vi "util_sort_build_specs.vi"(8 "error in (no error)":errorcluster, 11 "build_specifications in":T1[](array[typedef])) -> (0 "error out":errorcluster, 3 "build_specifications out":T1[](array[typedef]))   [LabVIEW 2015, in "lv-build.lvlib"]
uses:
  lv-build.lvlib
  public/_controls/build_specification.ctl
  public/_controls/build_type.ctl
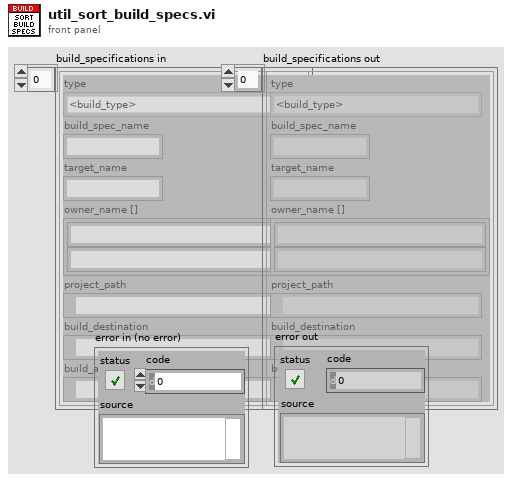
[diagram p1: front panel]
types:
  T1 = typedef "lv-build.lvlib/build_specification.ctl" = cluster{"type":T2, "build_spec_name":string, "target_name":string, "owner_name []":string[], "project_path":path, "build_destination":path, "build_artifact":path}
  T2 = typedef "lv-build.lvlib/build_type.ctl" = enum16{"<build_type>", "application_pc", "application_rt", "installer", "llb", "lvlibp", "zip", "fpga", "<null>"}
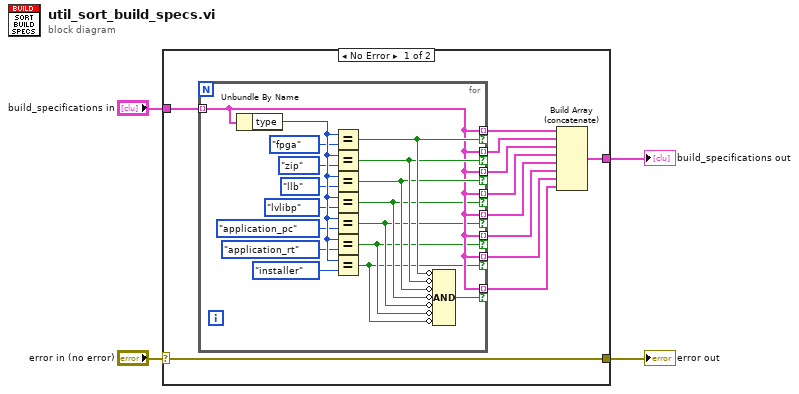
[diagram p0: block diagram]
diagram:
  n1 = case shown="No Error" "error in (no error)" {
    selector: "error in (no error)" -> [w11 w34]
    tunnel: "build_specifications in" -> [w15 w33]
    tunnel: [w12 w33] -> w3
    tunnel: [w11 w34] -> w1
    frame No Error {
      n2 = for {
        tunnel: w15 -> [w28] mode=indexing
        tunnel: [w28] -> w14 mode=indexing if=w31
        tunnel: [w28] -> w5 mode=indexing if=w32
        tunnel: [w28] -> w13 mode=indexing if=w30
        tunnel: [w28] -> w10 mode=indexing if=w29
        tunnel: [w28] -> w9 mode=indexing if=w26
        tunnel: [w28] -> w8 mode=indexing if=w25
        tunnel: [w28] -> w7 mode=indexing if=w24
        tunnel: [w28] -> w6 mode=indexing if=w23
        n3 = Unbundle By Name(w28) -> ("type"=w27:T2)
        n4 = Equal?(x=w27, y=build_type."fpga" ("Type")) -> (x = y?=w31:bool)
        n5 = Equal?(x=w27, y=build_type."zip" ("Type")) -> (x = y?=w30:bool)
        n6 = Equal?(x=w27, y=build_type."llb" ("Type")) -> (x = y?=w29:bool)
        n7 = Equal?(x=w27, y=build_type."lvlibp" ("Type")) -> (x = y?=w26:bool)
        n8 = Equal?(x=w27, y=build_type."application_pc" ("Type")) -> (x = y?=w25:bool)
        n9 = Equal?(x=w27, y=build_type."application_rt" ("Type")) -> (x = y?=w24:bool)
        n10 = Equal?(x=w27, y=build_type."installer" ("Type")) -> (x = y?=w23:bool)
        n11 = Compound Arithmetic op=AND(invert w31, invert w30, invert w29, invert w26, invert w25, invert w24, invert w23) -> (w32:bool)
      }
      n12 = Build Array (concatenate)(w14, w13, w10, w9, w8, w7, w6, w5) -> (w12:T1[])
    }
    frame Error {
    }
  }
  "build_specifications out" <- w3
  "error out" <- w1
